vi "HFRR ADV v03 new software.vi"() -> ()   [LabVIEW 2025] (continued)
                n1294 = property on="ENTER THE NEW PASSWORD" class="Str"("Visible"=FALSE) -> ()  [unwired: 2 in, 2 out]
              }
              frame True {
                # "password"
                # "change password logic"
                n1295 = local read "ENTER CURRENT PASSWORD"() -> (w2276:string)
                n1296 = local read "dipl pwd"() -> (w2270:string)
                n1297 = String To Byte Array(string=w2276) -> (unsigned byte array=w2278:u8[])
                n1298 = String To Byte Array(string=w2270) -> (unsigned byte array=w2271:u8[])
                n1299 = Array Size(array=w2278) -> (size(s)=w2275:i32)
                n1300 = Array Size(array=w2271) -> (size(s)=w2273:i32)
                n1301 = for {
                  N: w2275 -> [_]
                  tunnel: w2278 -> [w2302]
                  tunnel: [w2300] -> w2279 mode=indexing
                  tunnel: w2275 -> [w2294]
                  i -> [w2295]
                  n1302 = Decrement(x=w2294) -> (x-1=w2292:i32)
                  n1303 = Equal?(x=w2295, y=w2292) -> (x = y?=w2293:bool)
                  n1304 = Index Array(array=w2302, index=w2295) -> (element=w2296:u8)
                  n1305 = Number To Decimal String(number=w2296) -> (decimal integer string=w2301:string)  [unwired: 1 in]
                  n1306 = Select(t="", s=w2293, f="\r") -> (s? t:f=w2298:string)
                  n1307 = Concatenate Strings(w2301, w2298) -> (w2300:string)
                }
                n1308 = for {
                  N: w2273 -> [_]
                  tunnel: w2271 -> [w2290]
                  tunnel: [w2288] -> w2272 mode=indexing
                  tunnel: w2273 -> [w2285]
                  i -> [w2286]
                  n1309 = Decrement(x=w2285) -> (x-1=w2284:i32)
                  n1310 = Equal?(x=w2286, y=w2284) -> (x = y?=w2283:bool)
                  n1311 = Index Array(array=w2290, index=w2286) -> (element=w2289:u8)
                  n1312 = Number To Decimal String(number=w2289) -> (decimal integer string=w2287:string)  [unwired: 1 in]
                  n1313 = Select(t="", s=w2283, f="\r") -> (s? t:f=w2280:string)
                  n1314 = Concatenate Strings(w2287, w2280) -> (w2288:string)
                }
                n1315 = local read "string"() -> (w2277:string)
                n1316 = Concatenate Strings(w2272) -> (w2266:string)
                n1317 = Concatenate Strings(w2277) -> (w2274:string)
                n1318 = Concatenate Strings(w2279) -> (w2267:string)
                n1319 = Equal?(x=w2267, y=w2274) -> (x = y?=w2269:bool)
                n1320 = Equal?(x=w2267, y=w2266) -> (x = y?=w2265:bool)
                n1321 = Or(x=w2269, y=w2265) -> (x .or. y?=w2268:bool)
                n1322 = case shown="True" w2268 {
                  frame False {
                  }
                  frame True {
                    n1323 = property on="ENTER THE NEW PASSWORD" class="Str"("Visible"=TRUE) -> ()  [unwired: 2 in, 2 out]
                  }
                }
              }
            }
          }
          frame #2 {
            n1324 = String To Byte Array(string="ENTER THE NEW PASSWORD") -> (unsigned byte array=w2305:u8[])
            n1325 = Search 1D Array(1D array=w2305, element=u8 10) -> (index of element=w2309:i32)  [unwired: 1 in]
            n1326 = Index Array(array=w2305, index=w2309) -> (element=w2307:u8)
            n1327 = Equal?(x=w2307, y=10) -> (x = y?=w2304:bool)
            n1328 = case shown="False" w2304 {
              frame False {
              }
              frame True {
                n1329 = local write "EDIT"(FALSE) -> ()
                n1330 = local write "SrvM CP"(FALSE) -> ()
                n1331 = local read "ENTER THE NEW PASSWORD"() -> (w2312:string)
                n1332 = String To Byte Array(string=w2312) -> (unsigned byte array=w2317:u8[])
                n1333 = Array Size(array=w2317) -> (size(s)=w2314:i32)
                n1334 = for {
                  N: w2314 -> [_]
                  tunnel: w2317 -> [w2330]
                  tunnel: [w2327] -> w2319 mode=indexing
                  tunnel: w2314 -> [w2322]
                  i -> [w2320]
                  n1335 = Decrement(x=w2322) -> (x-1=w2323:i32)
                  n1336 = Equal?(x=w2320, y=w2323) -> (x = y?=w2324:bool)
                  n1337 = Index Array(array=w2330, index=w2320) -> (element=w2329:u8)
                  n1338 = Number To Decimal String(number=w2329) -> (decimal integer string=w2328:string)  [unwired: 1 in]
                  n1339 = Select(t="", s=w2324, f="\r") -> (s? t:f=w2321:string)
                  n1340 = Concatenate Strings(w2328, w2321) -> (w2327:string)
                }
                n1341 = local read "file path"() -> (w2311:path)
                n1342 = Concatenate Strings(w2319) -> (w2313:string)
                n1343 = Delete(path (use dialog)=w2311) -> (deleted path=w2315:path)  [unwired: 4 in, 2 out]
                n1344 = call <vilib>:"Write Characters To File.vi"("append to file? (new file:F)"=FALSE, "character string"=w2313, "file path (dialog if empty)"=w2315) -> ()  [unwired: 2 in, 1 out]
              }
            }
          }
          frame #3 {
            n1345 = case shown="True" "SrvM CP" {
              frame False {
                w2333 = ""
                n1346 = local write "ENTER CURRENT PASSWORD"(w2333) -> ()
                n1347 = local write "ENTER THE NEW PASSWORD"(w2333) -> ()
                n1348 = property on="ENTER CURRENT PASSWORD" class="Str"("Visible"=FALSE) -> ()  [unwired: 2 in, 2 out]
              }
              frame True {
                n1349 = property on="ENTER THE NEW PASSWORD" class="Str"() -> ("Visible"=w2334:bool)  [unwired: 2 in, 2 out]
                n1350 = Not(x=w2334) -> (.not. x?=w2335:bool)
                n1351 = property on="ENTER CURRENT PASSWORD" class="Str"("Visible"=w2335) -> ()  [unwired: 2 in, 2 out]
              }
            }
          }
          frame #4 {
            n1352 = String To Byte Array(string="Password") -> (unsigned byte array=w2342:u8[])
            n1353 = Search 1D Array(1D array=w2342, element=u8 10) -> (index of element=w2340:i32)  [unwired: 1 in]
            n1354 = Index Array(array=w2342, index=w2340) -> (element=w2341:u8)
            n1355 = Equal?(x=w2341, y=10) -> (x = y?=w2337:bool)
            n1356 = case shown="True" w2337 {
              frame False {
              }
              frame True {
                # "password"
                # "password"
                n1357 = local read "Password"() -> (w2355:string)
                n1358 = String To Byte Array(string=w2355) -> (unsigned byte array=w2358:u8[])
                n1359 = String To Byte Array(string="@143$\n") -> (unsigned byte array=w2344:u8[])
                n1360 = Array Size(array=w2358) -> (size(s)=w2353:i32)
                n1361 = Array Size(array=w2344) -> (size(s)=w2349:i32)
                n1362 = for {
                  N: w2353 -> [_]
                  tunnel: w2358 -> [w2392]
                  tunnel: [w2390] -> w2359 mode=indexing
                  tunnel: w2353 -> [w2387]
                  i -> [w2388]
                  n1363 = Decrement(x=w2387) -> (x-1=w2386:i32)
                  n1364 = Index Array(array=w2392, index=w2388) -> (element=w2391:u8)
                  n1365 = Equal?(x=w2388, y=w2386) -> (x = y?=w2385:bool)
                  n1366 = Number To Decimal String(number=w2391) -> (decimal integer string=w2389:string)  [unwired: 1 in]
                  n1367 = Select(t="", s=w2385, f="\r") -> (s? t:f=w2382:string)
                  n1368 = Concatenate Strings(w2389, w2382) -> (w2390:string)
                }
                n1369 = for {
                  N: w2349 -> [_]
                  tunnel: w2344 -> [w2403]
                  tunnel: [w2401] -> w2347 mode=indexing
                  tunnel: w2349 -> [w2398]
                  i -> [w2399]
                  n1370 = Decrement(x=w2398) -> (x-1=w2397:i32)
                  n1371 = Index Array(array=w2403, index=w2399) -> (element=w2402:u8)
                  n1372 = Equal?(x=w2399, y=w2397) -> (x = y?=w2396:bool)
                  n1373 = Number To Decimal String(number=w2402) -> (decimal integer string=w2400:string)  [unwired: 1 in]
                  n1374 = Select(t="", s=w2396, f="\r") -> (s? t:f=w2393:string)
                  n1375 = Concatenate Strings(w2400, w2393) -> (w2401:string)
                }
                n1376 = local read "file path"() -> (w2343:path)
                n1377 = call <vilib>:"Read Characters From File.vi"("file path (dialog if empty)"=w2343) -> ("character string"=w2357:string)  [unwired: 5 in, 3 out]
                "string" <- w2357
                n1378 = flat-sequence {
                  tunnel: [w2360] -> w2354
                  frame #0 {
                    w2360 = ""
                    n1379 = local write "Password"(w2360) -> ()
                  }
                }
                n1380 = Concatenate Strings(w2347) -> (w2348:string)
                n1381 = Concatenate Strings(w2357) -> (w2356:string)
                n1382 = Concatenate Strings(w2359) -> (w2351:string)
                n1383 = Equal?(x=w2351, y=w2356) -> (x = y?=w2346:bool)
                n1384 = Equal?(x=w2351, y=w2348) -> (x = y?=w2352:bool)
                n1385 = Or(x=w2346, y=w2352) -> (x .or. y?=w2345:bool)
                "x = y?" <- w2345
                n1386 = case shown="True" w2345 {
                  selector: w2345 -> [w2362 _]
                  tunnel: w2354 -> [_ _]
                  frame False {
                    n1387 = And(x=w2362, y=TRUE ("Visible")) -> (x .and. y?=w2363:bool)
                    n1388 = property on="message" class="Str"("Visible"=w2363) -> ()  [unwired: 2 in, 2 out]
                  }
                  frame True {
                    n1389 = control-ref of="This VI"() -> (w2374:refnum<vi>)
                    n1390 = property class="VI"(reference=w2374) -> (reference out=w2365:refnum<vi>, error out=w2369:errorcluster, "Panel"=w2373:refnum<vi>)  [unwired: 1 in]
                    n1391 = property on="message" class="Str"("Visible"=FALSE) -> ()  [unwired: 2 in, 2 out]
                    n1392 = property class="Pnl"(reference=w2373, error in=w2369) -> (reference out=w2367:refnum<vi>, error out=w2370:errorcluster, "Panes[]"=w2372:refnum<vi>[])
                    n1393 = for {
                      tunnel: w2372 -> [w2381] mode=indexing
                      tunnel: T15."Always On" ("Horizontal Scrollbar Visibility") -> [w2380]
                      tunnel: w2370 -> [w2377]
                      tunnel: [w2376] -> w2368
                      n1394 = property class="Pane"(reference=w2381, error in=w2377, "HorizScrollbarVisibility"=w2380) -> (reference out=w2378:refnum<vi>, error out=w2379:errorcluster)
                      n1395 = Close Reference(reference=w2378, error in (no error)=w2379) -> (error out=w2376:errorcluster)
                    }
                    n1396 = Close Reference(reference=w2367, error in (no error)=w2368) -> (error out=w2366:errorcluster)
                    n1397 = Close Reference(reference=w2365, error in (no error)=w2366) -> (error out=→"error out 6":errorcluster)
                  }
                }
              }
            }
          }
        }
        n1398 = local read "x = y?"() -> (w2202:bool)
        n1399 = local read "HUMIDITY: 2"() -> (w2204:dbl)
        n1400 = local read "HUMIDITY:"() -> (w2203:dbl)
        n1401 = property on="Port 2 Error" class="Clust (strict)"("Visible"="EDIT") -> ()  [unwired: 2 in, 2 out]
        n1402 = property on="Port 1 Error" class="Clust (strict)"("Visible"="EDIT") -> ()  [unwired: 2 in, 2 out]
        n1403 = case shown="True" "SrvM CP 2" {
          frame False {
          }
          frame True {
            n1404 = local write "SrvM CP 2"(FALSE ("SrvM CP 2")) -> ()
            n1405 = local read "HUMIDITY: 2"() -> (w2243:dbl)
            n1406 = local read "TEMP INTERCEPT: 2"() -> (w2242:dbl)
            n1407 = local read "DISPLACEMENT : 4"() -> (w2246:dbl)
            n1408 = local read "TEMPERATURE : 2"() -> (w2245:dbl)
            n1409 = local read "STROKE GAIN : 2"() -> (w2247:dbl)
            n1410 = local read "FRIC. FORCE : 2"() -> (w2248:dbl)
            n1411 = local read "AIR TEMP INTERCEPT: 2"() -> (w2241:dbl)
            n1412 = local read "AIR TEMPERATURE : 2"() -> (w2244:dbl)
            n1413 = local write "HUMIDITY:"(w2243) -> ()
            n1414 = local write "AIR TEMP INTERCEPT:"(w2242) -> ()
            n1415 = local write "TEMPERATURE :"(w2245) -> ()
            n1416 = local write "FRIC. FORCE :"(w2248) -> ()
            n1417 = local write "STROKE GAIN :"(w2247) -> ()
            n1418 = local write "DISPLACEMENT :"(w2246) -> ()
            n1419 = local write "AIR TEMPERATURE :"(w2244) -> ()
            n1420 = local write "TEMP INTERCEPT:"(w2241) -> ()
          }
        }
        n1421 = Or(x="SAVE", y=w2196) -> (x .or. y?=w2197:bool)
        n1422 = And(x="EDIT", y=w2202) -> (x .and. y?=w2200:bool)
        n1423 = local read "DISPLACEMENT : 4"() -> (w2213:dbl)
        n1424 = local read "TEMPERATURE : 2"() -> (w2211:dbl)
        n1425 = local read "STROKE GAIN : 2"() -> (w2217:dbl)
        n1426 = local read "DISPLACEMENT :"() -> (w2212:dbl)
        n1427 = local read "FRIC. FORCE : 2"() -> (w2220:dbl)
        n1428 = local read "TEMPERATURE :"() -> (w2209:dbl)
        n1429 = local read "STROKE GAIN :"() -> (w2216:dbl)
        n1430 = local read "FRIC. FORCE :"() -> (w2219:dbl)
        n1431 = case shown="True" w2200 {
          tunnel: [u8 2 ("Disabled") u8 0 ("Disabled")] -> w2199
          tunnel: [w2564 TRUE ("Visible")] -> w2198
          frame False {
            w2564 = FALSE ("Visible")
            n1432 = local write "EDIT 2"(w2564) -> ()
          }
          frame True {
          }
        }
        n1433 = case shown="True" w2197 {
          frame False {
          }
          frame True {
            n1434 = stacked-sequence {
              seq-local: [w2412 _ _] -> [_ w2559 _]
              frame #0 {
                (unwired) i16 5 ("precision (6)")
                # "[CH1]    - FF\n[CH2]   - TEMPERATURE\n[CH3]    - Humidity\n[CH4]    - AIR TEMP\n[CH5]\\- Visa Uno\n[CH6] \\- Visa Due\n[CH7]  \\- file path\n[CH8]   - Displacement Gain\n[CHA]   - Stroke Gain\n[CHB]   - Stroke PID Gain\n[CHC]   -Language Selection\n[CHD]   -Power +\n[CHE]   -Power_\n[CHF]   -Heater\n[CHG]   -Humidity Wet\n[CHH]   -Humidity Dry\n[CHI]   -Integral Time"
                n1435 = local read "Language Selection"() -> (w2460:enum16{"English", "Russian"})
                n1436 = local read "CH-HUMIDITY WET"() -> (w2418:u16)
                n1437 = local read "CH-HUMIDITY DRY"() -> (w2415:u16)
                n1438 = local read "STROKE GAIN :"() -> (w2404:dbl)
                n1439 = local read "CH-POWER +"() -> (w2427:u16)
                n1440 = local read "CH-POWER -"() -> (w2424:u16)
                n1441 = local read "CH-HEATER"() -> (w2421:u16)
                n1442 = local read "AIR TEMPERATURE :"() -> (w2407:dbl)
                n1443 = local read "DISPLACEMENT :"() -> (w2405:dbl)
                n1444 = local read "TEMPERATURE :"() -> (w2408:dbl)
                n1445 = local read "FRIC. FORCE :"() -> (w2409:dbl)
                n1446 = local read "HUMIDITY:"() -> (w2406:dbl)
                n1447 = Path To String(path="File Path") -> (string=w2476:string)
                n1448 = Number To Fractional String(number=w2404, width (-)=i16 10 ("precision (6)"), precision (6)=i16 5) -> (F-format string=w2467:string)  [unwired: 1 in]
                n1449 = Number To Fractional String(number=w2460, width (-)=i16 10 ("precision (6)"), precision (6)=i16 5) -> (F-format string=w2456:string)  [unwired: 1 in]
                n1450 = Number To Fractional String(number=w2427, width (-)=i16 10 ("precision (6)"), precision (6)=i16 5) -> (F-format string=w2450:string)  [unwired: 1 in]
                n1451 = Number To Fractional String(number=w2424, width (-)=i16 10 ("precision (6)"), precision (6)=i16 5) -> (F-format string=w2447:string)  [unwired: 1 in]
                n1452 = Number To Fractional String(number=w2421, width (-)=i16 10 ("precision (6)"), precision (6)=i16 5) -> (F-format string=w2442:string)  [unwired: 1 in]
                n1453 = Number To Fractional String(number=w2418, width (-)=i16 10 ("precision (6)"), precision (6)=i16 5) -> (F-format string=w2439:string)  [unwired: 1 in]
                n1454 = Number To Fractional String(number=w2415, width (-)=i16 10 ("precision (6)"), precision (6)=i16 5) -> (F-format string=w2434:string)  [unwired: 1 in]
                n1455 = local read "Com Port 1"() -> (w2411:refnum<visa-resource-name>)
                n1456 = local read "Com Port 2"() -> (w2410:refnum<visa-resource-name>)
                n1457 = Concatenate Strings(w2476, "\\" ("string")) -> (w2475:string)
                n1458 = Number To Fractional String(number=w2409, width (-)=i16 10 ("precision (6)"), precision (6)=i16 5) -> (F-format string=w2508:string)  [unwired: 1 in]
                n1459 = Number To Fractional String(number=w2408, width (-)=i16 10 ("precision (6)"), precision (6)=i16 5) -> (F-format string=w2507:string)  [unwired: 1 in]
                n1460 = Number To Fractional String(number=w2406, width (-)=i16 10 ("precision (6)"), precision (6)=i16 5) -> (F-format string=w2501:string)  [unwired: 1 in]
                n1461 = Number To Fractional String(number=w2407, width (-)=i16 10 ("precision (6)"), precision (6)=i16 5) -> (F-format string=w2495:string)  [unwired: 1 in]
                n1462 = Number To Fractional String(number=w2405, width (-)=i16 10 ("precision (6)"), precision (6)=i16 5) -> (F-format string=w2468:string)  [unwired: 1 in]
                n1463 = Concatenate Strings("[CHA]" ("string"), w2467, "- Stroke Gain" ("string"), "\r") -> (w2461:string)
                n1464 = Concatenate Strings("[CHC]" ("string"), w2456, "-Language Selection" ("string"), "\r") -> (w2453:string)
                n1465 = Concatenate Strings("[CHD]" ("string"), w2450, "-Power +" ("string"), "\r") -> (w2432:string)
                n1466 = Concatenate Strings("[CHG]" ("string"), w2439, "-Humidity Wet" ("string"), "\r") -> (w2429:string)
                n1467 = Concatenate Strings("[CHH]" ("string"), w2434, "-Humidity Dry" ("string"), "\r") -> (w2428:string)
                n1468 = Concatenate Strings("[CH1]" ("string"), w2508, " - FF" ("string"), "\r") -> (w2506:string)
                n1469 = Concatenate Strings("[CH2]" ("string"), w2507, " - TEMPERATURE" ("string"), "\r") -> (w2505:string)
                n1470 = Concatenate Strings("[CH3]" ("string"), w2501, " - Humidity" ("string"), "\r") -> (w2498:string)
                n1471 = Concatenate Strings("[CH4]" ("string"), w2495, " - AIR TEMP" ("string"), "\r") -> (w2491:string)
                n1472 = Concatenate Strings("[CH5]" ("string"), w2411, "- Visa Uno" ("string"), "\r") -> (w2484:string)
                n1473 = Concatenate Strings("[CH6]" ("string"), w2410, "- Visa Due" ("string"), "\r") -> (w2479:string)
                n1474 = Concatenate Strings("[CH7]" ("string"), w2475, "- file path" ("string"), "\r") -> (w2478:string)
                n1475 = Concatenate Strings("[CH8]" ("string"), w2468, "- Displacement Gain" ("string"), "\r") -> (w2471:string)
                n1476 = Concatenate Strings("[CHE]" ("string"), w2447, "-Power_" ("string"), "\r") -> (w2431:string)
                n1477 = Concatenate Strings("[CHF]" ("string"), w2442, "-Heater" ("string"), "\r") -> (w2430:string)
                n1478 = Concatenate Strings(w2506, w2505, w2498, w2491, w2484, w2479, w2478, w2471, w2461, w2453, w2432, w2431, w2430, w2429, w2428) -> (w2412:string)
                "gain" <- w2412
              }
              frame #1 {
                n1479 = local read "Camera Port :"() -> (w2520:string)
                n1480 = local read "C3 :"() -> (w2528:refnum<visa-resource-name>)
                n1481 = local read "TEMP INTERCEPT:"() -> (w2529:dbl)
                n1482 = local read "AIR TEMP INTERCEPT:"() -> (w2530:dbl)
                n1483 = Concatenate Strings("[CH8]" ("string"), w2520, "- Visa Camera" ("string"), "\r") -> (w2519:string)
                n1484 = Concatenate Strings("[CH7]" ("string"), w2528, "- Visa Humidity" ("string"), "\r") -> (w2524:string)
                n1485 = Number To Fractional String(number=w2529, width (-)=i16 10 ("precision (6)"), precision (6)=i16 5) -> (F-format string=w2547:string)  [unwired: 1 in]
                n1486 = local read "Com Port 3"() -> (w2531:refnum<visa-resource-name>)
                n1487 = Number To Fractional String(number=w2530, width (-)=i16 10 ("precision (6)"), precision (6)=i16 5) -> (F-format string=w2554:string)  [unwired: 1 in]
                n1488 = Concatenate Strings("[CHK]" ("string"), w2547, "-TEMP INTERCEPT" ("string"), "\r") -> (w2543:string)
                n1489 = Concatenate Strings("[SNO]" ("string"), "S.NO", "-" ("string"), "\r") -> (w2539:string)
                n1490 = Concatenate Strings("[CHJ]" ("string"), w2554, "-AIR TEMP INTERCEPT" ("string"), "\r") -> (w2544:string)
                n1491 = Concatenate Strings("[CHL]" ("string"), w2531, "- Visa humid" ("string"), "\r") -> (w2534:string)
                n1492 = String To Path(string="C:\\LAB-IQ\\calibrate WO 2465.dcf") -> (path=w2532:path)
                n1493 = Concatenate Strings(w2559, w2544, w2543, w2539, w2534, w2524, w2519) -> (w2558:string)
                n1494 = call <vilib>:"Write Characters To File.vi"("append to file? (new file:F)"=FALSE, "character string"=w2558, "file path (dialog if empty)"=w2532) -> ()  [unwired: 2 in, 1 out]
              }
              frame #2 {
                n1495 = local write "Lan flag"(0.0 ("Lan flag")) -> ()
                n1496 = local write "conststatus"(0.0 ("rpm value : 2")) -> ()
                n1497 = local write "SAVE"(FALSE ("OK Button 14")) -> ()
                n1498 = local write "SAVE 2"(FALSE ("SAVE 2")) -> ()
              }
            }
          }
        }
        n1499 = Subtract(x=w2204, y=w2203) -> (x-y=w2205:dbl)
        n1500 = local read "AIR TEMPERATURE : 2"() -> (w2208:dbl)
        n1501 = local read "AIR TEMPERATURE :"() -> (w2207:dbl)
        n1502 = Divide(x=w2205, y=w2203) -> (x/y=w2227:dbl)
        n1503 = Subtract(x=w2220, y=w2219) -> (x-y=w2218:dbl)
        n1504 = Subtract(x=w2211, y=w2209) -> (x-y=w2210:dbl)
        n1505 = Subtract(x=w2217, y=w2216) -> (x-y=w2215:dbl)
        n1506 = Subtract(x=w2213, y=w2212) -> (x-y=w2214:dbl)
        n1507 = Subtract(x=w2208, y=w2207) -> (x-y=w2206:dbl)
        n1508 = Divide(x=w2218, y=w2219) -> (x/y=w2238:dbl)
        n1509 = Divide(x=w2210, y=w2209) -> (x/y=w2231:dbl)
        n1510 = Divide(x=w2215, y=w2216) -> (x/y=w2235:dbl)
        n1511 = Divide(x=w2214, y=w2212) -> (x/y=w2234:dbl)
        n1512 = Multiply(x=w2227, y=100.0) -> (x*y=→"HUMIDITY  Calibration Error":dbl)
        n1513 = Divide(x=w2206, y=w2207) -> (x/y=w2230:dbl)
        n1514 = Multiply(x=w2238, y=100.0) -> (x*y=→"FRIC. FORCE Calibration Error":dbl)
        n1515 = Multiply(x=w2231, y=100.0) -> (x*y=→"TEMPERATURE  Calibration Error":dbl)
        n1516 = Multiply(x=w2235, y=100.0) -> (x*y=→"STROKE Calibration Error":dbl)
        n1517 = Multiply(x=w2234, y=100.0) -> (x*y=→"DISPLACEMENT  Calibration Error":dbl)
        n1518 = property on="EDIT 2" class="Bool (strict)"("Visible"=w2198) -> ()  [unwired: 2 in, 2 out]
        n1519 = property on="SAVE" class="Bool (strict)"("Visible"=w2198) -> ()  [unwired: 2 in, 2 out]
        n1520 = property on="SrvM CP" class="Bool (strict)"("Disabled"=w2199) -> ()  [unwired: 2 in, 2 out]
        n1521 = property on="visa due" class="CmbBox"("Disabled"=w2199) -> ()  [unwired: 2 in, 2 out]
        n1522 = property on="File Path" class="Path"("Disabled"=w2199) -> ()  [unwired: 2 in, 2 out]
        n1523 = Multiply(x=w2230, y=100.0) -> (x*y=→"AIR TEMPERATURE  Calibration Error":dbl)
        n1524 = property on="Language Selection" class="Enum (strict)"("Visible"=w2198) -> ()  [unwired: 2 in, 2 out]
        n1525 = property on="Tab Control 7" class="TabCtl (strict)"("Disabled"=w2199) -> ()  [unwired: 2 in, 2 out]
        n1526 = property on="AIR TEMP INTERCEPT:" class="DigNum (strict)"("Disabled"=w2199) -> ()  [unwired: 2 in, 2 out]
        n1527 = property on="CH-POWER -" class="DigNum (strict)"("Disabled"=w2199) -> ()  [unwired: 2 in, 2 out]
        n1528 = property on="CH-POWER +" class="DigNum (strict)"("Disabled"=w2199) -> ()  [unwired: 2 in, 2 out]
        n1529 = property on="AIR TEMPERATURE :" class="DigNum (strict)"("Disabled"=w2199) -> ()  [unwired: 2 in, 2 out]
        n1530 = property on="STROKE GAIN :" class="DigNum (strict)"("Disabled"=w2199) -> ()  [unwired: 2 in, 2 out]
        n1531 = property on="SPEED OUT:" class="DigNum (strict)"("Disabled"=w2199) -> ()  [unwired: 2 in, 2 out]
        n1532 = property on="CH-HUMIDITY DRY" class="DigNum (strict)"("Disabled"=w2199) -> ()  [unwired: 2 in, 2 out]
        n1533 = property on="HUMIDITY:" class="DigNum (strict)"("Disabled"=w2199) -> ()  [unwired: 2 in, 2 out]
        n1534 = property on="CH-HUMIDITY WET" class="DigNum (strict)"("Disabled"=w2199) -> ()  [unwired: 2 in, 2 out]
        n1535 = property on="TEMPERATURE :" class="DigNum (strict)"("Disabled"=w2199) -> ()  [unwired: 2 in, 2 out]
        n1536 = property on="DISPLACEMENT :" class="DigNum (strict)"("Disabled"=w2199) -> ()  [unwired: 2 in, 2 out]
        n1537 = property on="CH-HEATER" class="DigNum (strict)"("Disabled"=w2199) -> ()  [unwired: 2 in, 2 out]
        n1538 = property on="TEMP INTERCEPT:" class="DigNum (strict)"("Disabled"=w2199) -> ()  [unwired: 2 in, 2 out]
        n1539 = property on="FRIC. FORCE :" class="DigNum (strict)"("Disabled"=w2199) -> ()  [unwired: 2 in, 2 out]
      }
    }
    n1540 = local read "RUN"() -> (w1593:bool)
    n1541 = local read "RUN"() -> (w1591:bool)
    n1542 = disable-structure shown="Disabled" {
      disable-tunnel: [w1608 _] -> w1574
      disable-tunnel: [w1607 _] -> w1572
      frame Disabled {
        n1543 = local read "Temperature before test"() -> (w1601:dbl)
        n1544 = local read "Temperature after test"() -> (w1614:dbl)
        n1545 = case shown="True" "Save Results" {
          frame False {
          }
          frame True {
            w1630 = "\r"
            n1546 = local write "Save Results"(FALSE ("OK Button 5")) -> ()
            n1547 = local read "Temperature before test"() -> (w1668:dbl)
            n1548 = local read "Temperature after test"() -> (w1670:dbl)
            n1549 = local read "Humidity before test"() -> (w1667:dbl)
            n1550 = local read "Humidity after test"() -> (w1669:dbl)
            n1551 = local read "WS1.4"() -> (w1674:dbl)
            n1552 = local read "AVP"() -> (w1672:dbl)
            n1553 = Number To Fractional String(number=w1674, width (-)=i16 6, precision (6)=i16 1) -> (F-format string=w1634:string)  [unwired: 1 in]
            n1554 = local read "MWSD"() -> (w1671:dbl)
            n1555 = local read "String"() -> (w1663:string)
            n1556 = local read "FILE"() -> (w1666:string)
            n1557 = local read "HCF"() -> (w1673:dbl)
            n1558 = Number To Fractional String(number=w1667, width (-)=i16 6, precision (6)=i16 1) -> (F-format string=w1659:string)  [unwired: 1 in]
            n1559 = Number To Fractional String(number=w1668, width (-)=i16 6, precision (6)=i16 1) -> (F-format string=w1656:string)  [unwired: 1 in]
            n1560 = Number To Fractional String(number=w1669, width (-)=i16 6, precision (6)=i16 1) -> (F-format string=w1652:string)  [unwired: 1 in]
            n1561 = Number To Fractional String(number=w1670, width (-)=i16 6, precision (6)=i16 1) -> (F-format string=w1648:string)  [unwired: 1 in]
            n1562 = Number To Fractional String(number=w1672, width (-)=i16 6, precision (6)=i16 3) -> (F-format string=w1641:string)  [unwired: 1 in]
            n1563 = Concatenate Strings(w1663, w1666) -> (w1685:string)
            n1564 = Number To Fractional String(number=w1671, width (-)=i16 6, precision (6)=i16 1) -> (F-format string=w1645:string)  [unwired: 1 in]
            n1565 = Number To Fractional String(number=w1673, width (-)=i16 6, precision (6)=i16 2) -> (F-format string=w1639:string)  [unwired: 1 in]
            n1566 = Concatenate Strings("(" ("string"), w1634, ")Microns" ("string")) -> (w1633:string)
            n1567 = local read "REMARKS"() -> (w1665:string)
            "REMARKS 2" <- w1665
            n1568 = Concatenate Strings("(" ("string"), w1659, " ) % RH," ("string")) -> (w1660:string)
            n1569 = Concatenate Strings(w1639, ")" ("string")) -> (w1637:string)
            n1570 = Concatenate Strings("(" ("string"), w1656, ")  Deg C ," ("string")) -> (w1655:string)
            n1571 = Concatenate Strings("(" ("string"), w1652, " ) % RH," ("string")) -> (w1651:string)
            n1572 = Concatenate Strings("(" ("string"), w1648, ")  Deg C ," ("string")) -> (w1647:string)
            n1573 = Concatenate Strings("(" ("string"), w1645, ")  Microns," ("string")) -> (w1644:string)
            n1574 = Concatenate Strings("(" ("string"), w1641, ")  kPa," ("string")) -> (w1631:string)
            n1575 = Concatenate Strings(w1685, ".dwm" ("Substring")) -> (w1683:string)
            n1576 = String To Path(string=w1683) -> (path=w1682:path)
            n1577 = Concatenate Strings(w1665, w1630, " Humidity before test= " ("Substring"), w1660, w1630, " Temperature before test = " ("Substring"), w1655, w1630, " Humidity after test= " ("Substring"), w1651, w1630, "Temperature after test = " ("Substring"), w1647, w1630, "MSD = " ("Substring"), w1644, w1630, "  AVP = " ("Substring"), w1631, w1630, "  HCF                     =( " ("Substring"), w1637, w1630, " WS1.4                  = " ("Substring"), w1633, w1630) -> (w1629:string)
            "data" <- w1629
            n1578 = call <vilib>:"Write Characters To File.vi"("append to file? (new file:F)"=FALSE, "character string"=w1629, "file path (dialog if empty)"=w1682) -> ()  [unwired: 2 in, 1 out]
            n1579 = Match Pattern(string=w1629, regular expression="!") -> (after substring=→"export":string)  [unwired: 1 in, 3 out]
          }
        }
        n1580 = Add(x=231.864, y=w1601) -> (x+y=w1598:dbl)
        n1581 = Add(x=231.864, y=w1614) -> (x+y=w1611:dbl)
        n1582 = Divide(x=1705.984, y=w1598) -> (x/y=w1599:dbl)
        n1583 = Divide(x=1705.984, y=w1611) -> (x/y=w1612:dbl)
        n1584 = local read "Humidity before test"() -> (w1603:dbl)
        n1585 = local read "Humidity after test"() -> (w1616:dbl)
        n1586 = Subtract(x=8.017352 ("y"), y=w1599) -> (x-y=w1625:dbl)
        n1587 = Subtract(x=8.017352 ("y"), y=w1612) -> (x-y=w1619:dbl)
        n1588 = expression code="10**y"(w1625) -> (w1605:dbl)
        n1589 = expression code="10**y"(w1619) -> (w1618:dbl)
        n1590 = Multiply(x=w1603, y=w1605) -> (x*y=w1604:dbl)
        n1591 = Multiply(x=w1616, y=w1618) -> (x*y=w1617:dbl)
        n1592 = Divide(x=w1604, y=750.0) -> (x/y=w1620:dbl)
        n1593 = Divide(x=w1617, y=750.0) -> (x/y=w1621:dbl)
        n1594 = Add(x=w1620, y=w1621) -> (x+y=w1622:dbl)
        n1595 = Divide(x=w1622, y=2.0) -> (x/y=w1624:dbl)
        n1596 = local write "AVP"(w1624) -> ()
        n1597 = Subtract(x=1.4, y=w1624) -> (x-y=w1607:dbl)
        n1598 = local read "HCF"() -> (w1608:dbl)
      }
      frame Enabled {
      }
    }
    n1599 = case shown="True" "EDIT 3" {
      frame False {
      }
      frame True {
        n1600 = local write "EDIT 3"(FALSE ("EDIT 3")) -> ()
        n1601 = local write "Main Tab"(T2."About" ("Main Tab")) -> ()
      }
    }
    n1602 = case shown="False" w1593 {
      frame False {
        n1603 = local read "stopT"() -> (w2571:bool)
        n1604 = case shown="True" w2571 {
          frame False {
          }
          frame True {
            n1605 = local write "stopT"(FALSE) -> ()
          }
        }
      }
      frame True {
        "stopT" <- TRUE
      }
    }
    n1606 = case shown="False" w1591 {
      frame False {
      }
      frame True {
      }
    }
    n1607 = case shown="True" w1581 {
      frame False {
        n1608 = property on="Password 2" class="Str"("Visible"=FALSE) -> ()  [unwired: 2 in, 2 out]
        n1609 = local write "Password 2"("" ("Password")) -> ()
      }
      frame True {
        n1610 = property on="Password 2" class="Str"("Visible"=TRUE) -> ()  [unwired: 2 in, 2 out]
        n1611 = Equal?(x="Password 2", y="HFRR1234") -> (x = y?=w1713:bool)
        n1612 = case shown="True" w1713 {
          tunnel: "Password 2" -> [w1716 _]
          frame False {
            n1613 = String Length(string=w1716) -> (length=w1717:i32)
            n1614 = Greater Than 0?(x=w1717) -> (x > 0?=w1715:bool)
            n1615 = case shown="False" w1715 {
              frame False {
                n1616 = property on="Password 2" class="Str"("Caption.Text"="Password (Advance Setting)") -> ()  [unwired: 2 in, 2 out]
              }
              frame True {
                n1617 = property on="Password 2" class="Str"("Caption.Text"="Incorrect Password!") -> ()  [unwired: 2 in, 2 out]
              }
            }
          }
          frame True {
            n1618 = local write "EDIT 2"(FALSE ("EDIT 2")) -> ()
            n1619 = local write "Password 2"("" ("Password")) -> ()
            n1620 = local write "Main Tab"(T2."Advance" ("Main Tab")) -> ()
            n1621 = local write "Main Dashboard Buttons"(T1."Advance" ("Main Dashboard Buttons")) -> ()
          }
        }
      }
    }
    n1622 = case shown="True" "Prog Uno" {
      frame False {
      }
      frame True {
        n1623 = stacked-sequence {
          frame #0 {
            n1624 = Delete(path (use dialog)=path "C:/LAB-IQ-NXT/UNOCOMPILE.bat" ("working directory")) -> ()  [unwired: 4 in, 3 out]
          }
          frame #1 {
            n1625 = local read "Com Port 1"() -> (w2178:refnum<visa-resource-name>)
            n1626 = Concatenate Strings("cmd.exe /c \"mode " ("command line"), w2178, ":1200,n,8,1\"\n" ("command line")) -> (w2183:string)
            n1627 = Concatenate Strings(w2183, "CD\\\nCD WinDucom\navrdude -C avrdude.conf -v -patmega328p -carduino -P" ("command line"), w2178, " -b115200 -D -Uflash:w:UNO_V20.hex:i\n" ("command line"), "\r") -> (w2185:string)
            "STR" <- w2185
            n1628 = call <vilib>:"Write Characters To File.vi"("append to file? (new file:F)"=FALSE, "character string"=w2185, "file path (dialog if empty)"=path "C:/LAB-IQ/UNOCOMPILE.bat" ("working directory")) -> ()  [unwired: 2 in, 1 out]
          }
          frame #2 {
            n1629 = disable-structure shown="Disabled" {
              frame Disabled {
                w2189 = "cmd.exe  /c \"C:\\LAB-IQ-NXT\\UNOCOMPILE.bat\"" ("string")
                n1630 = local write "Prog Uno"(FALSE ("run minimized? (F)")) -> ()
                n1631 = call <vilib>:"System Exec.vi"("expected output size  (4096)"=u32 65535, "run minimized? (F)"=FALSE, "wait until completion? (T)"=TRUE ("run minimized? (F)"), "working directory"=path "C:/LAB-IQ-NXT", "standard input"=w2189, "command line"=w2189) -> ("error out"=w2188:errorcluster, "standard output"=→"String 42":string)  [unwired: 2 in, 2 out]
                "error out 3" <- w2188
                n1632 = flat-sequence {
                  tunnel: w2188 -> [_]
                  frame #0 {
                  }
                }
              }
              frame Enabled {
              }
            }
          }
        }
      }
    }
    n1633 = case shown="\"CEC F-096-A-06\"" "TEST STANDARD" {
      tunnel: [2.0 ("Set Temp") 0.0 ("Set Temp") 2.0 ("Set Temp") 0.0 ("Set Temp")] -> w1582
      frame "ASTM D6079", Default {
        w2135 = 50.0 ("Hz")
        w2136 = 53.0 ("Set Rh")
        w2138 = 1.0 ("Set Strk")
        w2137 = 60.0 ("Set Temp")
        # "astm hide"
        n1634 = local write "NORMAL LOAD"(200.0 ("NORMAL LOAD")) -> ()
        n1635 = local write "Set Strk"(w2138) -> ()
        n1636 = local write "Set Hz"(w2135) -> ()
        n1637 = local write "Set Temp"(w2137) -> ()
        n1638 = local write "Set Rh"(w2136) -> ()
        n1639 = local write "test time"(75.0 ("test time")) -> ()
        n1640 = local write "Set Stroke:"(w2138) -> ()
        n1641 = local write "Set Humidity:"(w2136) -> ()
        n1642 = local write "Set Frequency:"(w2135) -> ()
        n1643 = local write "Set Temperature:"(w2137) -> ()
        "Test Standard" <- "ASTM D6079" ("Test Standard 2")
      }
      frame "ISO 12156" {
        n1644 = local write "Set Strk"(1.0 ("Set Strk")) -> ()
        n1645 = local write "NORMAL LOAD"(200.0 ("NORMAL LOAD")) -> ()
        n1646 = local write "Set Temp"(60.0 ("Set Temp")) -> ()
        n1647 = local write "test time"(75.0 ("test time")) -> ()
        n1648 = local write "Set Hz"(50.0 ("Hz")) -> ()
        n1649 = local write "Set Rh"(53.0 ("Set Rh")) -> ()
      }
      frame "CEC F-096-A-06" {
        n1650 = local write "Set Strk"(1.0 ("Set Strk")) -> ()
        n1651 = local write "NORMAL LOAD"(200.0 ("NORMAL LOAD")) -> ()
        n1652 = local write "Set Temp"(60.0 ("Set Temp")) -> ()
        n1653 = local write "test time"(75.0 ("test time")) -> ()
        n1654 = local write "Set Hz"(50.0 ("Hz")) -> ()
        n1655 = local write "Set Rh"(53.0 ("Set Rh")) -> ()
      }
      frame "Custom" {
      }
    }
    n1656 = case shown="True" "Prog Due" {
      frame False {
      }
      frame True {
        n1657 = stacked-sequence {
          frame #0 {
            n1658 = Delete(path (use dialog)=path "C:/LAB-IQ/DUECOMPILE.bat" ("working directory")) -> ()  [unwired: 4 in, 3 out]
          }
          frame #1 {
            n1659 = disable-structure shown="Disabled" {
              frame Disabled {
                n1660 = local read "visa due"() -> (w2160:string)
                n1661 = Concatenate Strings("cmd.exe /c \"mode " ("command line"), w2160, ":1200,n,8,1\"\n" ("command line")) -> (w2165:string)
                n1662 = Concatenate Strings(w2165, "CD\\\nCD WinDucom\nTIMEOUT 1\n bossac.exe -i -d --port=" ("command line"), w2160, " -U false -e -w -v -b DUE.bin -R\n" ("command line"), "\r") -> (w2167:string)
                "concatenated string 2" <- w2167
                n1663 = call <vilib>:"Write Characters To File.vi"("append to file? (new file:F)"=FALSE, "character string"=w2167, "file path (dialog if empty)"=path "C:/LAB-IQ-NXT/DUECOMPILE.bat" ("working directory")) -> ()  [unwired: 2 in, 1 out]
              }
              frame Enabled {
              }
            }
          }
          frame #2 {
            # "C:\\LAB-IQ-NXT\\DUECOMPILE.bat"
            n1664 = disable-structure shown="Disabled" {
              frame Disabled {
                w2172 = "cmd.exe  /c \"C:\\LAB-IQ-NXT\\DUECOMPILE.bat\"" ("string")
                n1665 = call <vilib>:"System Exec.vi"("expected output size  (4096)"=u32 65535, "run minimized? (F)"=FALSE, "wait until completion? (T)"=TRUE ("run minimized? (F)"), "working directory"=path "C:/LAB-IQ-NXT", "standard input"=w2172, "command line"=w2172) -> ("error out"=w2171:errorcluster, "standard output"=→"String 44":string)  [unwired: 2 in, 2 out]
                "error out 4" <- w2171
                n1666 = flat-sequence {
                  tunnel: w2171 -> [_]
                  frame #0 {
                  }
                }
              }
              frame Enabled {
              }
            }
            n1667 = local write "Prog Due"(FALSE ("Prog Due")) -> ()
          }
        }
      }
    }
    n1668 = Or(x=w1579, y=w1577) -> (x .or. y?=w1578:bool)
    n1669 = case shown="\"About\"" w1576 {
      tunnel: [T20."Acquire" ("Main Tab") T20."Compare Files" ("Main Tab") T20."About" ("Main Tab")] -> w1589
      frame "Acquire", Default {
      }
      frame "Compare Files" {
      }
      frame "About" {
      }
    }
    n1670 = Or(x=w1583, y="OPEN") -> (x .or. y?=w1584:bool)
    n1671 = case shown="True" w1584 {
      tunnel: w1583 -> [_ w1724]
      frame False {
      }
      frame True {
        n1672 = stacked-sequence {
          tunnel: w1724 -> [_ w1791 _ _]
          frame #0 {
            w1740 = "  " ("String 6")
            n1673 = local write "OPEN"(FALSE ("open")) -> ()
            n1674 = local read "string1 2"() -> (w1728:string)
            n1675 = local read "string1 3"() -> (w1727:string)
            n1676 = local read "string1 4"() -> (w1726:string)
            n1677 = property on="OPEN" class="Bool (strict)"("Visible"=FALSE) -> ()  [unwired: 2 in, 2 out]
            n1678 = local write "String 6"(w1740) -> ()
            n1679 = local write "String 7"(w1740) -> ()
            n1680 = local write "String 8"(w1740) -> ()
            n1681 = local write "String 12"(w1740) -> ()
            n1682 = local read "OK Button 16"() -> (w1725:bool)
            n1683 = String To Path(string=w1728) -> (path=w1736:path)
            n1684 = String To Path(string=w1727) -> (path=w1735:path)
            n1685 = String To Path(string=w1726) -> (path=w1734:path)
            n1686 = case shown="True" w1725 {
              tunnel: [w1741 w1742] -> w1729
              frame False {
                n1687 = local read "string1"() -> (w1741:string)
              }
              frame True {
                n1688 = local read "String Indicator 4"() -> (w1742:string)
              }
            }
            n1689 = Open/Create/Replace File "Open File"(file path (use dialog)=w1736) -> (refnum out=w1732:refnum<file>)  [unwired: 5 in, 2 out]
            n1690 = Open/Create/Replace File "Open File"(file path (use dialog)=w1735) -> (refnum out=w1731:refnum<file>)  [unwired: 5 in, 2 out]
            n1691 = Open/Create/Replace File "Open File"(file path (use dialog)=w1734) -> (refnum out=w1730:refnum<file>)  [unwired: 5 in, 2 out]
            n1692 = while {
              tunnel: w1732 -> [w1754]
              i -> [w1750]
              stop <- w1749 continue-if-true
              (unwired) TRUE ("line mode (F)")
              n1693 = Read from Text File "Read File"(file (use dialog)=w1754) -> (text=w1751:string)  [unwired: 3 in, 3 out]
              n1694 = local write "Numeric 11"(w1750) -> ()
              n1695 = String Length(string=w1751) -> (length=w1753:i32)
              n1696 = Greater?(x=w1753, y=1) -> (0:w1749:bool)
            }
            n1697 = while {
              tunnel: w1731 -> [w1760]
              i -> [w1756]
              stop <- w1755 continue-if-true
              (unwired) TRUE ("line mode (F)")
              n1698 = Read from Text File "Read File"(file (use dialog)=w1760) -> (text=w1757:string)  [unwired: 3 in, 3 out]
              n1699 = local write "Numeric 12"(w1756) -> ()
              n1700 = String Length(string=w1757) -> (length=w1759:i32)
              n1701 = Greater?(x=w1759, y=1) -> (0:w1755:bool)
            }
            n1702 = while {
              tunnel: w1730 -> [w1766]
              i -> [w1762]
              stop <- w1761 continue-if-true
              (unwired) TRUE ("line mode (F)")
              n1703 = Read from Text File "Read File"(file (use dialog)=w1766) -> (text=w1763:string)  [unwired: 3 in, 3 out]
              n1704 = local write "Numeric 13"(w1762) -> ()
              n1705 = String Length(string=w1763) -> (length=w1765:i32)
              n1706 = Greater?(x=w1765, y=1) -> (0:w1761:bool)
            }
            n1707 = String To Path(string=w1729) -> (path=w1737:path)
            n1708 = Open/Create/Replace File "Open File"(file path (use dialog)=w1737) -> (refnum out=w1733:refnum<file>)  [unwired: 5 in, 2 out]
            n1709 = while {
              tunnel: w1733 -> [w1748]
              i -> [w1744]
              stop <- w1743 continue-if-true
              (unwired) TRUE ("line mode (F)")
              n1710 = Read from Text File "Read File"(file (use dialog)=w1748) -> (text=w1745:string)  [unwired: 3 in, 3 out]
              n1711 = local write "Numeric 8"(w1744) -> ()
              n1712 = String Length(string=w1745) -> (length=w1747:i32)
              n1713 = Greater?(x=w1747, y=1) -> (0:w1743:bool)
            }
          }
          frame #1 {
            w1918 = FALSE ("ACTUAL   MERGE")
            # "Sample Temp"
            # "ECR"
            # "COF"
            # "Time\nCOF\nFF\nTemp"
            n1714 = case shown="True" w1791 {
              tunnel: [w1938 w1939] -> w1792
              frame False {
                n1715 = local read "string1"() -> (w1938:string)
              }
              frame True {
                n1716 = local read "String Indicator 4"() -> (w1939:string)
              }
            }
            n1717 = local read "string1 3"() -> (w1836:string)
            n1718 = String To Path(string=w1792) -> (path=w1923:path)
            n1719 = String To Path(string=w1836) -> (path=w1934:path)
            n1720 = local read "Numeric 12"() -> (w1920:i32)
            n1721 = local read "Numeric 8"() -> (w1922:i32)
            n1722 = local read "string1 2"() -> (w1837:string)
            n1723 = local read "string1 4"() -> (w1835:string)
            n1724 = Open/Create/Replace File "Open File"(file path (use dialog)=w1923) -> (refnum out=w1937:refnum<file>, error out=w1936:errorcluster)  [unwired: 5 in, 1 out]
            n1725 = Open/Create/Replace File "Open File"(file path (use dialog)=w1934) -> (refnum out=w1930:refnum<file>, error out=w1931:errorcluster)  [unwired: 5 in, 1 out]
            n1726 = for {
              N: w1922 -> [_]
              tunnel: w1937 -> [w2085]
              tunnel: w1936 -> [w2084]
              tunnel: [w2074] -> w1849 mode=indexing
              tunnel: [w2072] -> w1906 mode=indexing
              tunnel: [w2073] -> w1901 mode=indexing
              tunnel: w1918 -> [_]
              tunnel: [w2066] -> w1903 mode=indexing
              tunnel: [w2062] -> w1872 mode=indexing
              tunnel: [w2058] -> w1847 mode=indexing
              tunnel: [w2054] -> w1828 mode=indexing
              tunnel: [w2049] -> w1788 mode=indexing
              (unwired) TRUE ("line mode (F)")
              # "freq"
              # "Stroke"
              # "Time"
              # "CoF"
              # "Humidity"
              # "Temp"
              # "Air Temp"
              # "ECR"
              n1727 = Read from Text File "Read File"(file (use dialog)=w2085, error in=w2084) -> (text=w2050:string)  [unwired: 2 in, 3 out]
              n1728 = local write "String 6"(w2050) -> ()
              n1729 = String Subset(string=w2050, offset (0)=0, length (rest)=14 ("length (rest)")) -> (substring=w2078:string)
              n1730 = String Subset(string=w2050, offset (0)=35, length (rest)=9 ("length (rest)")) -> (substring=w2075:string)
              n1731 = String Subset(string=w2050, offset (0)=15, length (rest)=9 ("length (rest)")) -> (substring=w2081:string)
              n1732 = Fract/Exp String To Number(string=w2078) -> (number=w2074:dbl)  [unwired: 3 in, 1 out]
              n1733 = Fract/Exp String To Number(string=w2075) -> (number=w2073:dbl)  [unwired: 3 in, 1 out]
              n1734 = Fract/Exp String To Number(string=w2081) -> (number=w2072:dbl)  [unwired: 3 in, 1 out]
              n1735 = String Subset(string=w2050, offset (0)=85, length (rest)=9 ("length (rest)")) -> (substring=w2051:string)
              n1736 = String Subset(string=w2050, offset (0)=25, length (rest)=9 ("length (rest)")) -> (substring=w2057:string)
              n1737 = String Subset(string=w2050, offset (0)=55, length (rest)=9 ("length (rest)")) -> (substring=w2059:string)
              n1738 = String Subset(string=w2050, offset (0)=45, length (rest)=9 ("length (rest)")) -> (substring=w2065:string)
              n1739 = String Subset(string=w2050, offset (0)=65, length (rest)=9 ("length (rest)")) -> (substring=w2071:string)
              n1740 = Fract/Exp String To Number(string=w2057) -> (number=w2054:dbl)  [unwired: 3 in, 1 out]
              n1741 = Fract/Exp String To Number(string=w2051) -> (number=w2049:dbl)  [unwired: 3 in, 1 out]
              n1742 = Fract/Exp String To Number(string=w2059) -> (number=w2058:dbl)  [unwired: 3 in, 1 out]
              n1743 = Fract/Exp String To Number(string=w2065) -> (number=w2062:dbl)  [unwired: 3 in, 1 out]
              n1744 = Fract/Exp String To Number(string=w2071) -> (number=w2068:dbl)  [unwired: 3 in, 1 out]
              n1745 = Add(x=w2068, y=0.0) -> (x+y=w2066:dbl)
            }
            n1746 = for {
              N: w1920 -> [_]
              tunnel: w1931 -> [w2011]
              tunnel: w1930 -> [w2010]
              tunnel: [w2000] -> w1889 mode=indexing
              tunnel: [w1998] -> w1887 mode=indexing
              tunnel: [w1999] -> w1883 mode=indexing
              tunnel: w1918 -> [_]
              tunnel: [w1992] -> w1885 mode=indexing
              tunnel: [w1988] -> w1867 mode=indexing
              tunnel: [w1984] -> w1843 mode=indexing
              tunnel: [w1981] -> w1824 mode=indexing
              tunnel: [w1977] -> w1783 mode=indexing
              (unwired) 9 ("length (rest)")
              (unwired) 9 ("length (rest)")
              (unwired) TRUE ("line mode (F)")
              n1747 = Read from Text File "Read File"(file (use dialog)=w2010, error in=w2011) -> (text=w1978:string)  [unwired: 2 in, 3 out]
              n1748 = local write "String 8"(w1978) -> ()
              n1749 = String Subset(string=w1978, offset (0)=85) -> (substring=w1980:string)  [unwired: 1 in]
              n1750 = String Subset(string=w1978, offset (0)=35, length (rest)=9 ("length (rest)")) -> (substring=w2001:string)
              n1751 = String Subset(string=w1978, offset (0)=55, length (rest)=9 ("length (rest)")) -> (substring=w1986:string)
              n1752 = String Subset(string=w1978, offset (0)=25) -> (substring=w1982:string)  [unwired: 1 in]
              n1753 = String Subset(string=w1978, offset (0)=15, length (rest)=9 ("length (rest)")) -> (substring=w2007:string)
              n1754 = String Subset(string=w1978, offset (0)=0, length (rest)=14 ("length (rest)")) -> (substring=w2004:string)
              n1755 = String Subset(string=w1978, offset (0)=45, length (rest)=9 ("length (rest)")) -> (substring=w1991:string)
              n1756 = String Subset(string=w1978, offset (0)=65, length (rest)=9 ("length (rest)")) -> (substring=w1997:string)
              n1757 = Fract/Exp String To Number(string=w1980) -> (number=w1977:dbl)  [unwired: 3 in, 1 out]
              n1758 = Fract/Exp String To Number(string=w2001) -> (number=w1999:dbl)  [unwired: 3 in, 1 out]
              n1759 = Fract/Exp String To Number(string=w1986) -> (number=w1984:dbl)  [unwired: 3 in, 1 out]
              n1760 = Fract/Exp String To Number(string=w1982) -> (number=w1981:dbl)  [unwired: 3 in, 1 out]
              n1761 = Fract/Exp String To Number(string=w2007) -> (number=w1998:dbl)  [unwired: 3 in, 1 out]
              n1762 = Fract/Exp String To Number(string=w2004) -> (number=w2000:dbl)  [unwired: 3 in, 1 out]
              n1763 = Fract/Exp String To Number(string=w1991) -> (number=w1988:dbl)  [unwired: 3 in, 1 out]
              n1764 = Fract/Exp String To Number(string=w1997) -> (number=w1994:dbl)  [unwired: 3 in, 1 out]
              n1765 = Add(x=w1994, y=0.0) -> (x+y=w1992:dbl)
            }
            n1766 = String To Path(string=w1837) -> (path=w1935:path)
            n1767 = String To Path(string=w1835) -> (path=w1929:path)
            n1768 = local read "Numeric 11"() -> (w1919:i32)
            n1769 = local read "Numeric 13"() -> (w1921:i32)
            n1770 = Open/Create/Replace File "Open File"(file path (use dialog)=w1935) -> (refnum out=w1933:refnum<file>, error out=w1932:errorcluster)  [unwired: 5 in, 1 out]
            n1771 = Open/Create/Replace File "Open File"(file path (use dialog)=w1929) -> (refnum out=w1928:refnum<file>, error out=w1927:errorcluster)  [unwired: 5 in, 1 out]
            n1772 = for {
              N: w1919 -> [_]
              tunnel: w1933 -> [w2048]
              tunnel: w1932 -> [w2047]
              tunnel: [w2037] -> w1899 mode=indexing
              tunnel: [w2035] -> w1897 mode=indexing
              tunnel: [w2036] -> w1892 mode=indexing
              tunnel: w1918 -> [_]
              tunnel: [w2029] -> w1894 mode=indexing
              tunnel: [w2025] -> w1870 mode=indexing
              tunnel: [w2021] -> w1845 mode=indexing
              tunnel: [w2017] -> w1826 mode=indexing
              tunnel: [w2012] -> w1784 mode=indexing
              (unwired) TRUE ("line mode (F)")
              n1773 = Read from Text File "Read File"(file (use dialog)=w2048, error in=w2047) -> (text=w2013:string)  [unwired: 2 in, 3 out]
              n1774 = local write "String 7"(w2013) -> ()
              n1775 = String Subset(string=w2013, offset (0)=85, length (rest)=9 ("length (rest)")) -> (substring=w2016:string)
              n1776 = String Subset(string=w2013, offset (0)=35, length (rest)=9 ("length (rest)")) -> (substring=w2038:string)
              n1777 = String Subset(string=w2013, offset (0)=55, length (rest)=9 ("length (rest)")) -> (substring=w2024:string)
              n1778 = String Subset(string=w2013, offset (0)=25, length (rest)=9 ("length (rest)")) -> (substring=w2018:string)
              n1779 = String Subset(string=w2013, offset (0)=45, length (rest)=9 ("length (rest)")) -> (substring=w2026:string)
              n1780 = String Subset(string=w2013, offset (0)=0, length (rest)=14 ("length (rest)")) -> (substring=w2041:string)
              n1781 = String Subset(string=w2013, offset (0)=15, length (rest)=9 ("length (rest)")) -> (substring=w2044:string)
              n1782 = String Subset(string=w2013, offset (0)=65, length (rest)=9 ("length (rest)")) -> (substring=w2030:string)
              n1783 = Fract/Exp String To Number(string=w2016) -> (number=w2012:dbl)  [unwired: 3 in, 1 out]
              n1784 = Fract/Exp String To Number(string=w2038) -> (number=w2036:dbl)  [unwired: 3 in, 1 out]
              n1785 = Fract/Exp String To Number(string=w2024) -> (number=w2021:dbl)  [unwired: 3 in, 1 out]
              n1786 = Fract/Exp String To Number(string=w2018) -> (number=w2017:dbl)  [unwired: 3 in, 1 out]
              n1787 = Fract/Exp String To Number(string=w2026) -> (number=w2025:dbl)  [unwired: 3 in, 1 out]
              n1788 = Fract/Exp String To Number(string=w2041) -> (number=w2037:dbl)  [unwired: 3 in, 1 out]
              n1789 = Fract/Exp String To Number(string=w2044) -> (number=w2035:dbl)  [unwired: 3 in, 1 out]
              n1790 = Fract/Exp String To Number(string=w2030) -> (number=w2033:dbl)  [unwired: 3 in, 1 out]
              n1791 = Add(x=w2033, y=0.0) -> (x+y=w2029:dbl)
            }
            n1792 = for {
              N: w1921 -> [_]
              tunnel: w1928 -> [w1976]
              tunnel: w1927 -> [w1975]
              tunnel: [w1965] -> w1881 mode=indexing
              tunnel: [w1964] -> w1874 mode=indexing
              tunnel: w1918 -> [_]
              tunnel: [w1953] -> w1879 mode=indexing
              tunnel: [w1958] -> w1876 mode=indexing
              tunnel: [w1954] -> w1866 mode=indexing
              tunnel: [w1949] -> w1841 mode=indexing
              tunnel: [w1945] -> w1822 mode=indexing
              tunnel: [w1940] -> w1782 mode=indexing
              (unwired) 1.0 ("x")
              (unwired) TRUE ("line mode (F)")
              n1793 = Read from Text File "Read File"(file (use dialog)=w1976, error in=w1975) -> (text=w1941:string)  [unwired: 2 in, 3 out]
              n1794 = local write "String 12"(w1941) -> ()
              n1795 = String Subset(string=w1941, offset (0)=85, length (rest)=9 ("length (rest)")) -> (substring=w1943:string)
              n1796 = String Subset(string=w1941, offset (0)=35, length (rest)=9 ("length (rest)")) -> (substring=w1966:string)
              n1797 = String Subset(string=w1941, offset (0)=55, length (rest)=9 ("length (rest)")) -> (substring=w1951:string)
              n1798 = String Subset(string=w1941, offset (0)=25, length (rest)=9 ("length (rest)")) -> (substring=w1947:string)
